vi "Open References to Shared Variables.vi"(8 "error in (no error)":errorcluster, 10 "Process Data":T2={"Write URLs"={"URLs"=[], "Index DBL"=[], "Index Bool"=[]}, "Read URLs"={"URLs"=[], "Index DBL"=[], "Index Bool"=[]}, "Write SV FIFO"="", "Read SV FIFO"="", "Status Notifier"="", "Update Rate"=10}, 11 "SV Data":T1={"Status notifier"=refnum, "Write FIFO ref"=refnum, "Read FIFO ref"=refnum, "Update Rate"=1, "Write Refs by Type"={"DBL Write"=[], "Bool Write"=[], "DBLIndex"=[], "BoolIndex"=[]}, "Read Refs by Type"={"DBL Read"=[], "Bool Read"=[], "DBLIndex"=[], "BoolIndex"=[]}, "WriteSize"=0, "ReadSize"=0}) -> (0 "error out":errorcluster, 3 "SV Data":T1)   [LabVIEW 2016, in "Shared Variable Interface.lvlib"]
uses:
  Shared Variable Interface.lvlib
  Shared DataTypes/SV Process Data.ctl
  Shared DataTypes/URLs.ctl
  DataTypes/Bool.lvlib
  DataTypes/DBL.lvlib
panel:
  # "Out"
  # "In"
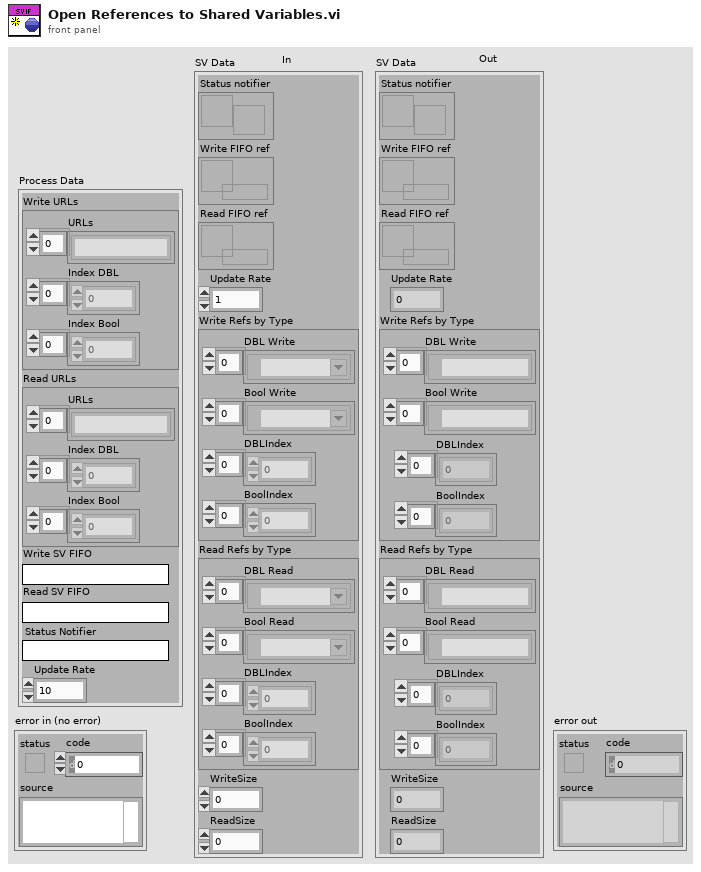
[diagram p1: front panel]
types:
  T1 = cluster{"Status notifier":refnum<notifier>, "Write FIFO ref":refnum<k33>, "Read FIFO ref":refnum<k33>, "Update Rate":u32, "Write Refs by Type":cluster{"DBL Write":refnum<k21>[], "Bool Write":refnum<k21>[], "DBLIndex":i32[], "BoolIndex":i32[]}, "Read Refs by Type":cluster{"DBL Read":refnum<k21>[], "Bool Read":refnum<k21>[], "DBLIndex":i32[], "BoolIndex":i32[]}, "WriteSize":i32, "ReadSize":i32}
  T2 = typedef "SV Process Data.ctl" = cluster{"Write URLs":T3, "Read URLs":T3, "Write SV FIFO":string, "Read SV FIFO":string, "Status Notifier":string, "Update Rate":u32}
  T3 = typedef "URLs.ctl" = cluster{"URLs":string[], "Index DBL":i32[], "Index Bool":i32[]}
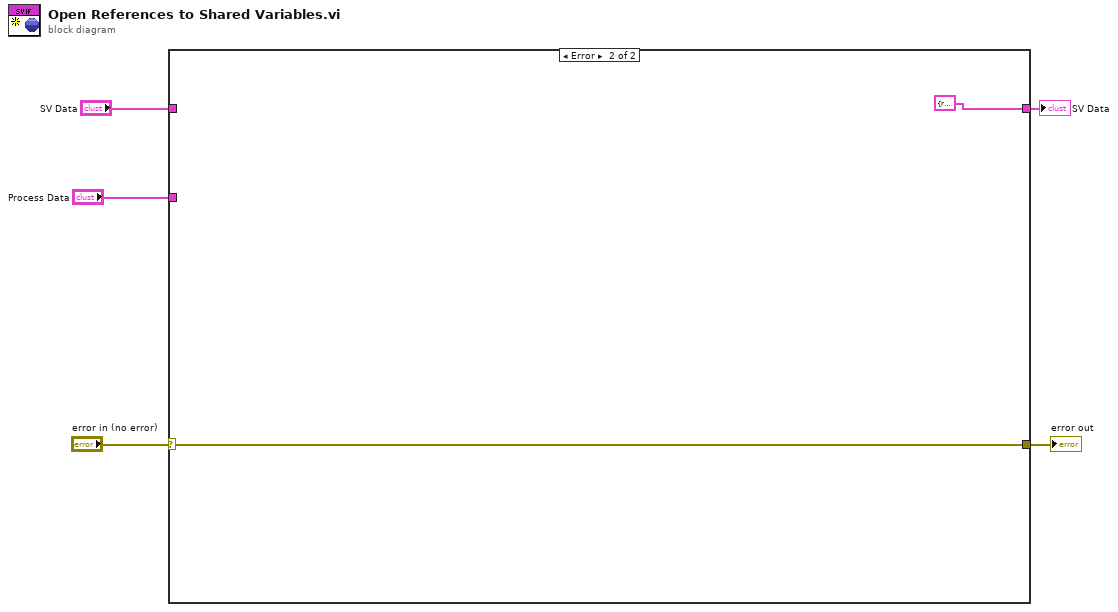
[diagram p0: block diagram]
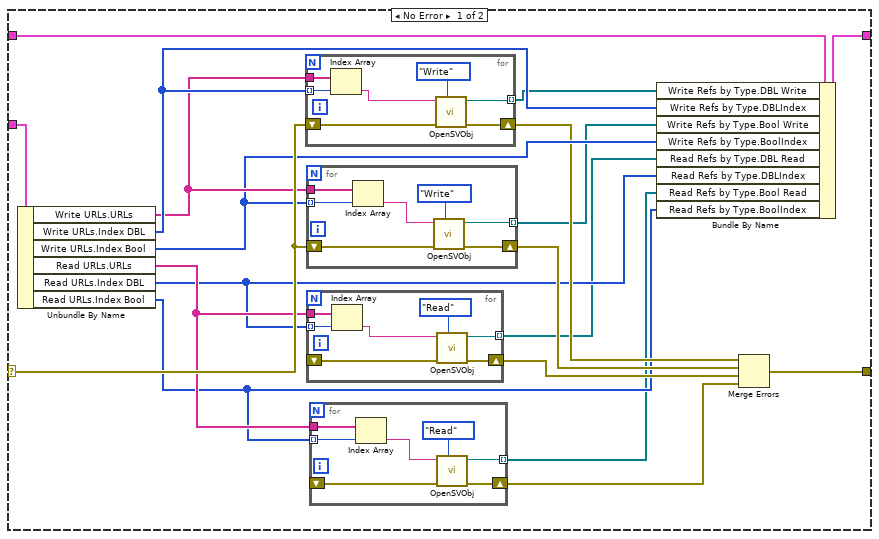
[diagram p2: hidden frame]
diagram:
  n1 = case shown="Error" "error in (no error)" {
    selector: "error in (no error)" -> [w20 w54]
    tunnel: [w24 w54] -> w4
    tunnel: [w22 T1 {"Status notifier"=refnum, "Write FIFO ref"=refnum, "Read FIFO ref"=refnum, "Update Rate"=0, "Write Refs by Type"={"DBL Write"=[], "Bool Write"=[], "DBLIndex"=[], "BoolIndex"=[]}, "Read Refs by Type"={"DBL Read"=[], "Bool Read"=[], "DBLIndex"=[], "BoolIndex"=[]}, "WriteSize"=0, "ReadSize"=0} ("SV Data")] -> w1
    tunnel: "Process Data" -> [w23 _]
    tunnel: "SV Data" -> [w6 _]
    frame No Error {
      n2 = Unbundle By Name(w23) -> ("Write URLs.URLs"=w19:string[], "Write URLs.Index DBL"=w21:i32[], "Write URLs.Index Bool"=w18:i32[], "Read URLs.URLs"=w13:string[], "Read URLs.Index DBL"=w11:i32[], "Read URLs.Index Bool"=w12:i32[])
      n3 = for {
        tunnel: w19 -> [w48]
        tunnel: [w52] -> w10 mode=indexing
        shift-right: [w51] -> w17
        shift-left: w20 -> [w50]
        tunnel: w21 -> [w49] mode=indexing
        n4 = Index Array(array=w48, index=w49) -> (element=w46:string)
        n5 = call "OpenSVObj.vi"("AccessType"=enum16{"Read", "Write"}."Write", "error in"=w50, "SVref"=w46) -> ("error out"=w51:errorcluster, "SVref"=w52:refnum<k21>)  [unwired: 7 in]
      }
      n6 = for {
        tunnel: w19 -> [w45]
        shift-right: [w39] -> w16
        shift-left: w20 -> [w40]
        tunnel: w18 -> [w44] mode=indexing
        tunnel: [w41] -> w9 mode=indexing
        n7 = Index Array(array=w45, index=w44) -> (element=w43:string)
        n8 = call "OpenSVObj.vi"("AccessType"=enum16{"Read", "Write"}."Write", "error in"=w40, "SVref"=w43) -> ("error out"=w39:errorcluster, "SV refnum"=w41:refnum<k21>)  [unwired: 7 in]
      }
      n9 = for {
        tunnel: w13 -> [w34]
        tunnel: [w38] -> w8 mode=indexing
        shift-right: [w37] -> w15
        shift-left: _ -> [w36]
        tunnel: w11 -> [w35] mode=indexing
        n10 = Index Array(array=w34, index=w35) -> (element=w32:string)
        n11 = call "OpenSVObj.vi"("AccessType"=enum16{"Read", "Write"}."Read", "error in"=w36, "SVref"=w32) -> ("error out"=w37:errorcluster, "SVref"=w38:refnum<k21>)  [unwired: 7 in]
      }
      n12 = for {
        tunnel: w13 -> [w31]
        shift-right: [w25] -> w14
        shift-left: _ -> [w26]
        tunnel: w12 -> [w30] mode=indexing
        tunnel: [w27] -> w7 mode=indexing
        n13 = Index Array(array=w31, index=w30) -> (element=w29:string)
        n14 = call "OpenSVObj.vi"("AccessType"=enum16{"Read", "Write"}."Read", "error in"=w26, "SVref"=w29) -> ("error out"=w25:errorcluster, "SV refnum"=w27:refnum<k21>)  [unwired: 7 in]
      }
      n15 = Bundle By Name(cluster=w6, "Write Refs by Type.DBL Write"=w10, "Write Refs by Type.DBLIndex"=w21, "Write Refs by Type.Bool Write"=w9, "Write Refs by Type.BoolIndex"=w18, "Read Refs by Type.DBL Read"=w8, "Read Refs by Type.DBLIndex"=w11, "Read Refs by Type.Bool Read"=w7, "Read Refs by Type.BoolIndex"=w12) -> (w22:T1)
      n16 = Merge Errors(w17, w16, w15, w14) -> (w24:errorcluster)
    }
    frame Error {
    }
  }
  "error out" <- w4
  "SV Data" <- w1
